vi "Dashboard Main.vi"() -> ()   [LabVIEW 2016]
uses:
  <vilib>/Utility/miscctls.llb/LVRowAndColumnTypeDef.ctl
  <vilib>/event_ctls.llb/eventvkey.ctl
  <vilib>/Rock Robotics/Network Tables/NT Read Numeric Array.vi
  <vilib>/Rock Robotics/Network Tables/NT Write Boolean.vi
  <vilib>/Rock Robotics/WPI/Dashboard/WPI_DashboardLogging Global.vi
panel:
  out "Camera Info 2":cluster{"Mbps LED":bool, "Mbps":dbl, "fps":dbl} {"fps" format="%#.1g"; "Mbps" format="%#.1g"}
  out "Background":bool
  out "Camera Image Right":T1(plugin-control)
  in  "Camera Settings Right":T2={"Frame Rate"=30, "Compression"=30, "Size"=1, "DB Camera Config"=FALSE} {"Frame Rate" scale=1.0..30.0; "Compression" scale=100.0..-1.0; "Size" items=["640x480", "320x240", "160x120"]}
  in  "Camera Name Right":string(combo)="No Camera Selection"
  out "Camera Info":cluster{"Mbps LED":bool, "Mbps":dbl, "fps":dbl} {"fps" format="%#.1g"; "Mbps" format="%#.1g"}
  in  "Camera Settings":T2={"Frame Rate"=30, "Compression"=30, "Size"=1, "DB Camera Config"=FALSE} {"Frame Rate" scale=1.0..30.0; "Compression" scale=100.0..-1.0; "Size" items=["640x480", "320x240", "160x120"]}
  in  "TCP":refnum<k5>
  in  "Rec Mode":enum32{"Stop", "Record", "Playback"}(radio)
  out "Robot IP":string
  out "Image Message":string="Timeout in Camera Communications"
  in  "Dashboard Tab":T3(tab)
  out "GEAR POSITION":string
  in  "Select Auto":string(combo)="Select Autonomous ..."
  out "NT Connection":bool
  out "MotorChart R":cluster{"Numeric":dbl, "Numeric":dbl}(graph)
  out "MotorChart L":cluster{"Numeric":dbl, "Numeric":dbl}(graph)
  out "MotorSliders R":cluster{"MotorSlide1":dbl, "MotorSlide2":dbl} {"MotorSlide2" scale=-1.0..1.0 scale format="%#_2e"; "MotorSlide1" scale=-1.0..1.0 scale format="%#_2e"}
  out "MotorSliders L":cluster{"MotorSlide1":dbl, "MotorSlide2":dbl} {"MotorSlide2" scale=-1.0..1.0 scale format="%#_2e"; "MotorSlide1" scale=-1.0..1.0 scale format="%#_2e"}
  out "Gyro":dbl(knob) scale=0.0..360.0
  out "JS1 Z":dbl(slide) scale=-1.0..1.0 scale format="%#_2e"
  out "JS1 Graph":cluster{"X":dbl, "Y":dbl}[](graph)
  out "JS1 Buttons":T4
  out "JS2 Z":dbl(slide) scale=-1.0..1.0 scale format="%#_2e"
  out "JS2 Graph":cluster{"X":dbl, "Y":dbl}[](graph)
  out "JS2 Buttons":T4
  out "Mode":T5(ring)=enum."Auto Disabled"
  in  "Drive Inverter":bool=TRUE
  in  "Turn Angle Target":dbl=30.0
  out "GEAR POSITION":dbl format="%#_13g"
  in  "Slow Speed":dbl(slide)=0.49999999999999994 scale=0.0..1.0
  out "Gyro Raw":dbl
  out "X-Axis Value":dbl=3.0 format="%#_13g"
  in  "D":dbl
  in  "I":dbl=10.0
  in  "Low":dbl=0.8
  in  "P":dbl=0.3
  in  "High":dbl=0.8
  in  "DB/String 9":string
  in  "DB/String 8":string
  in  "DB/String 7":string
  in  "DB/String 6":string
  in  "DB/String 5":string
  in  "DB/String 4":string
  in  "DB/String 3":string
  in  "DB/String 2":string
  in  "DB/String 1":string
  in  "DB/String 0":string
  in  "DB/Slider 0":dbl(slide) scale=0.0..5.0
  in  "DB/Slider 1":dbl(slide) scale=0.0..5.0
  in  "DB/Slider 2":dbl(slide) scale=0.0..5.0
  in  "DB/Slider 3":dbl(slide) scale=0.0..5.0
  out "DB/LED 3":bool
  out "DB/LED 2":bool
  out "DB/LED 1":bool
  out "DB/LED 0":bool
  in  "DB/Button 3":bool
  in  "DB/Button 2":bool
  in  "DB/Button 1":bool
  in  "DB/Button 0":bool caption="New Name"
  out "X-Axis Chart":dbl(graph)
  in  "T3":dbl=5.0
  in  "T2":dbl=2.0
  in  "T1":dbl=5.0
  in  "Y2":dbl=0.8
  in  "Y1":dbl=0.8
  in  "T4":dbl=3.0
  in  "X":dbl=-0.32
  in  "Y":dbl=0.8
  in  "Time":dbl=1.25
  in  "Gear Time":dbl=4.0
  in  "Time":dbl=1.0
  in  "Y 2":dbl=0.6
  in  "X 2":dbl=-0.32
  in  "Test Slider":dbl(slide) scale=0.0..100.0 scale format="%#_3g"
  in  "On/Off":bool caption="Solenoid"
  in  "Test Name":u16(ring) items=["Select the test to run..."]
  in  "Test Tree":string(tree)
  in  "Motor":cluster{"Value":dbl, "Enable":bool} {"Value" scale=-1.0..1.0 scale format="%#_3g"}
  out "Progress":T6 {"Test Progress" scale=0.0..100.0}
  in  "Rev/Fwd":cluster{"Forward":bool, "Reverse":bool}
  in  "Test Ring":u16(ring) items=["Monochrome", "Color"]
  out "Cmd Status":string
  in  "Execute Command":bool
  in  "Command Params":string[][](table)
  in  "Command Selection":i32(listbox)
  in  "CheckList":i32(listbox)
  out "Tree":string(tree)
  out "Camera Image":T1(plugin-control)
  in  "Camera Name":string(combo)="No Camera Selection"
  # "HW"
  # "HW"
  # "Joysticks"
  # "Drive Motors"
  # "Front"
  # "Right"
  # "Left"
  # "Back"
  # "POSITION 3 AUTON"
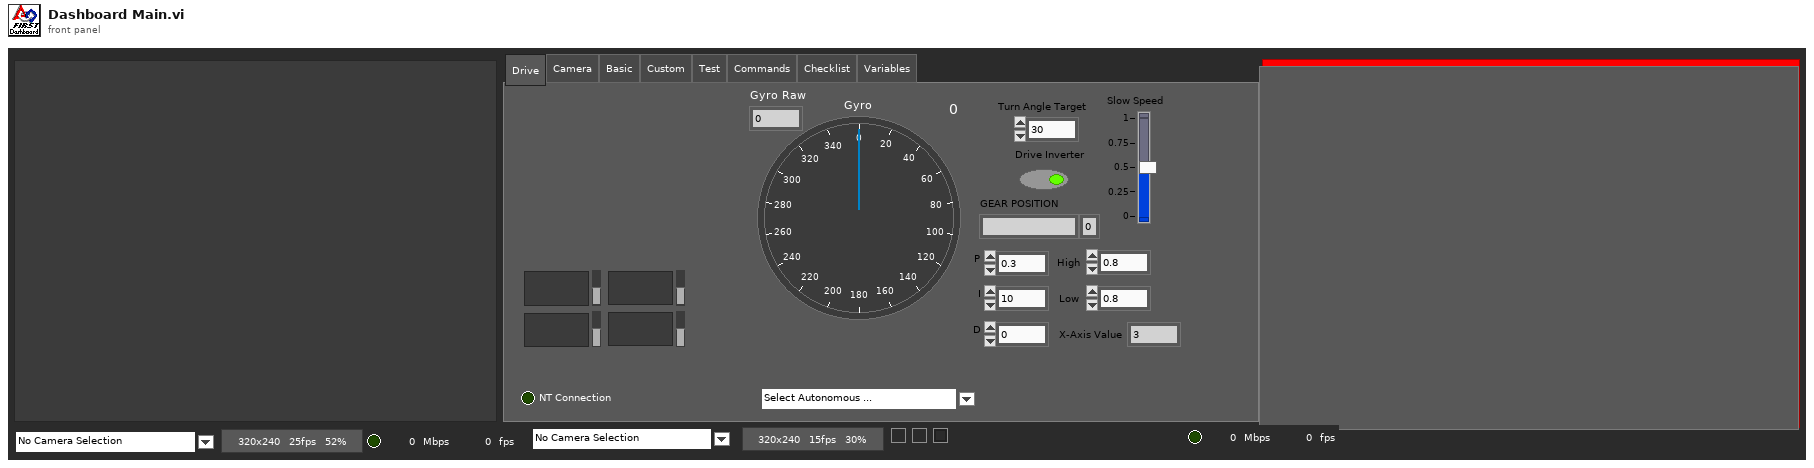
[diagram p1: front panel]
types:
  T1 = typedef "IMAQ Image.ctl" = refnum<image>
  T2 = cluster{"Frame Rate":i32, "Compression":i32, "Size":u16, "DB Camera Config":bool}
  T3 = enum32{"Drive", "Camera", "Basic", "Custom", "Test", "Commands", "Checklist", "Variables"}
  T4 = cluster{bool, bool, bool, bool, bool, bool, bool, bool, bool, bool, bool, bool}
  T5 = enum8{"Tele-Op Disabled", "Tele-Op Enabled", "Auto Disabled", "Auto Enabled", "Test Disabled", "Test Enabled", "Disconnected", "No Code", "E-Stop"}
  T6 = cluster{"Test Progress":u8, "Test Progress Text":string}
  T7 = typedef "Image Type" = u32
  T8 = cluster{"IDs":cluster{"RPC field ID":u16, "Unique ID":u16}, "String":string}
  T9 = enum32{"Drive", "Basic", "Custom", "Test", "Checklist", "Variables"}
  T10 = cluster{"Camera Image":refnum<vi>, "Dashboard Tab":refnum<vi>, "Background":refnum<vi>, "Rec Mode":refnum<vi>, "Test Slider":refnum<vi>, "On/Off ":refnum<vi>, "Test Ring":refnum<vi>, "Rev/Fwd":refnum<vi>, "Test Name":refnum<vi>, "Motor":refnum<vi>, "Progress":refnum<vi>, "CheckList":refnum<vi>, "Tree":refnum<vi>, "Test Tree":refnum<vi>, "Command Params":refnum<vi>, "Command Selection":refnum<vi>, "Execute Command":refnum<vi>, "Cmd Status":refnum<vi>, "Camera Settings":refnum<vi>, "Camera Name":refnum<vi>, "Camera Info":refnum<vi>, "Camera Settings Right":refnum<vi>, "Camera Name Right":refnum<vi>, "Camera Image Right":refnum<vi>}
  T11 = cluster{"Error Strings":string, "Disable Counts":cluster{u16, u16}, "Rail Faults":cluster{u16, u16, u16}, "Robot IP":string, "DB Mode":u8, "Event Info":cluster{"Name":string, "Type":u8, "Number":u16, "Replay":u8}}
  T12 = cluster{"Storage":cluster{"Disk Free":u64, "RAM Block":u32, "RAM free":u32}, "CPU Utilization":cluster{"CPU % ISR":sgl, "CPU % Time Crit":sgl, "CPU % Timed Str":sgl, "CPU % High":sgl, "CPU % Above":sgl, "CPU % Normal":sgl, "CPU % Low":sgl}, "CAN":cluster{"% Bus Utilization":sgl, "Bus Off Cnt":u32, "TX_FIFO Full Cnt":u32, "Receive Error Cnt":u8, "Transmit Error Cnt":u8}, "HID":cluster{"HID Outputs":u32, "Rumble Low":u16, "Rumble High":u16}[]}
  T13 = cluster{"Status bits":cluster{"Test Mode":bool, "Autonomous":bool, "Enabled":bool, "Code Start":bool, "Brownout":bool, "Reserved 2":bool, "Reserved 3":bool, "E-Stop":bool}, "Code Trace":cluster{"Disabled":bool, "TeleOp":bool, "Auto":bool, "Test":bool}, "Controller Type":enum16{"unknown", "cRIO", "roboRio"}, "Code?":enum16{"unknown", "noCode", "code"}, "Battery V":dbl}
  T14 = cluster{"Control Bits":cluster{"TestMode":bool, "Autonomous":bool, "Enabled":bool, "FMS Present":bool, bool, bool, bool, "E-Stop":bool}, "Team Station ":u8, "Countdown":sgl, "Joystick Values":cluster{"Axes":dbl[], "Buttons":bool[], "POVs":i16[]}[]}
  T15 = cluster{"Axes":dbl[], "Buttons":bool[], "POVs":i16[]}[]
  T16 = cluster{"Axes":dbl[], "Buttons":bool[], "POVs":i16[]}
  T17 = cluster{"Buttons[0]":bool, "Buttons[1]":bool, "Buttons[2]":bool, "Buttons[3]":bool, "Buttons[4]":bool, "Buttons[5]":bool, "Buttons[6]":bool, "Buttons[7]":bool, "Buttons[8]":bool, "Buttons[9]":bool, "Buttons[10]":bool, "Buttons[11]":bool}
  T18 = cluster{"Operation":enum16{"Update", "Clear"}, "Color Box":u32}[]
  T19 = typedef "eventvkey.ctl" = enum16{"ASCII", "Enter", "Return", "Shift", "Ctrl", "Alt", "Cmd", "Opt", "Caps", "NumLock", "Clear", "Break", "Up", "Down", "Left", "Right", "Insert", "Delete", "Home", "End", "PageUp", "PageDown", "Escape", "Help", "Pause", "ScrollLock", "F1", "F2", "F3", "F4", "F5", "F6", "F7", "F8", "F9", "F10", "F11", "F12", "F13", "F14", "F15", "F16", "F17", "F18", "F19", "F20", "F21", "F22", "F23", "F24", "Play", "VolumeUp", "VolumeDown", "Mute", "Two Byte Char"}
  T20 = cluster{"Image Size":bool, "Image Type":bool, "Pixel Value":bool, "ROI Information":bool, "Zoom Factor":bool}
  T21 = cluster{"Operation":enum16{"Update", "Clear"}, "Color Box":u32}
  T22 = typedef "LVRowAndColumnTypeDef.ctl" = cluster{"Row":i32, "Column":i32}
  T23 = cluster{"Shift":bool, "Ctrl":bool, "Alt":bool, "Cmd":bool, "Opt":bool}
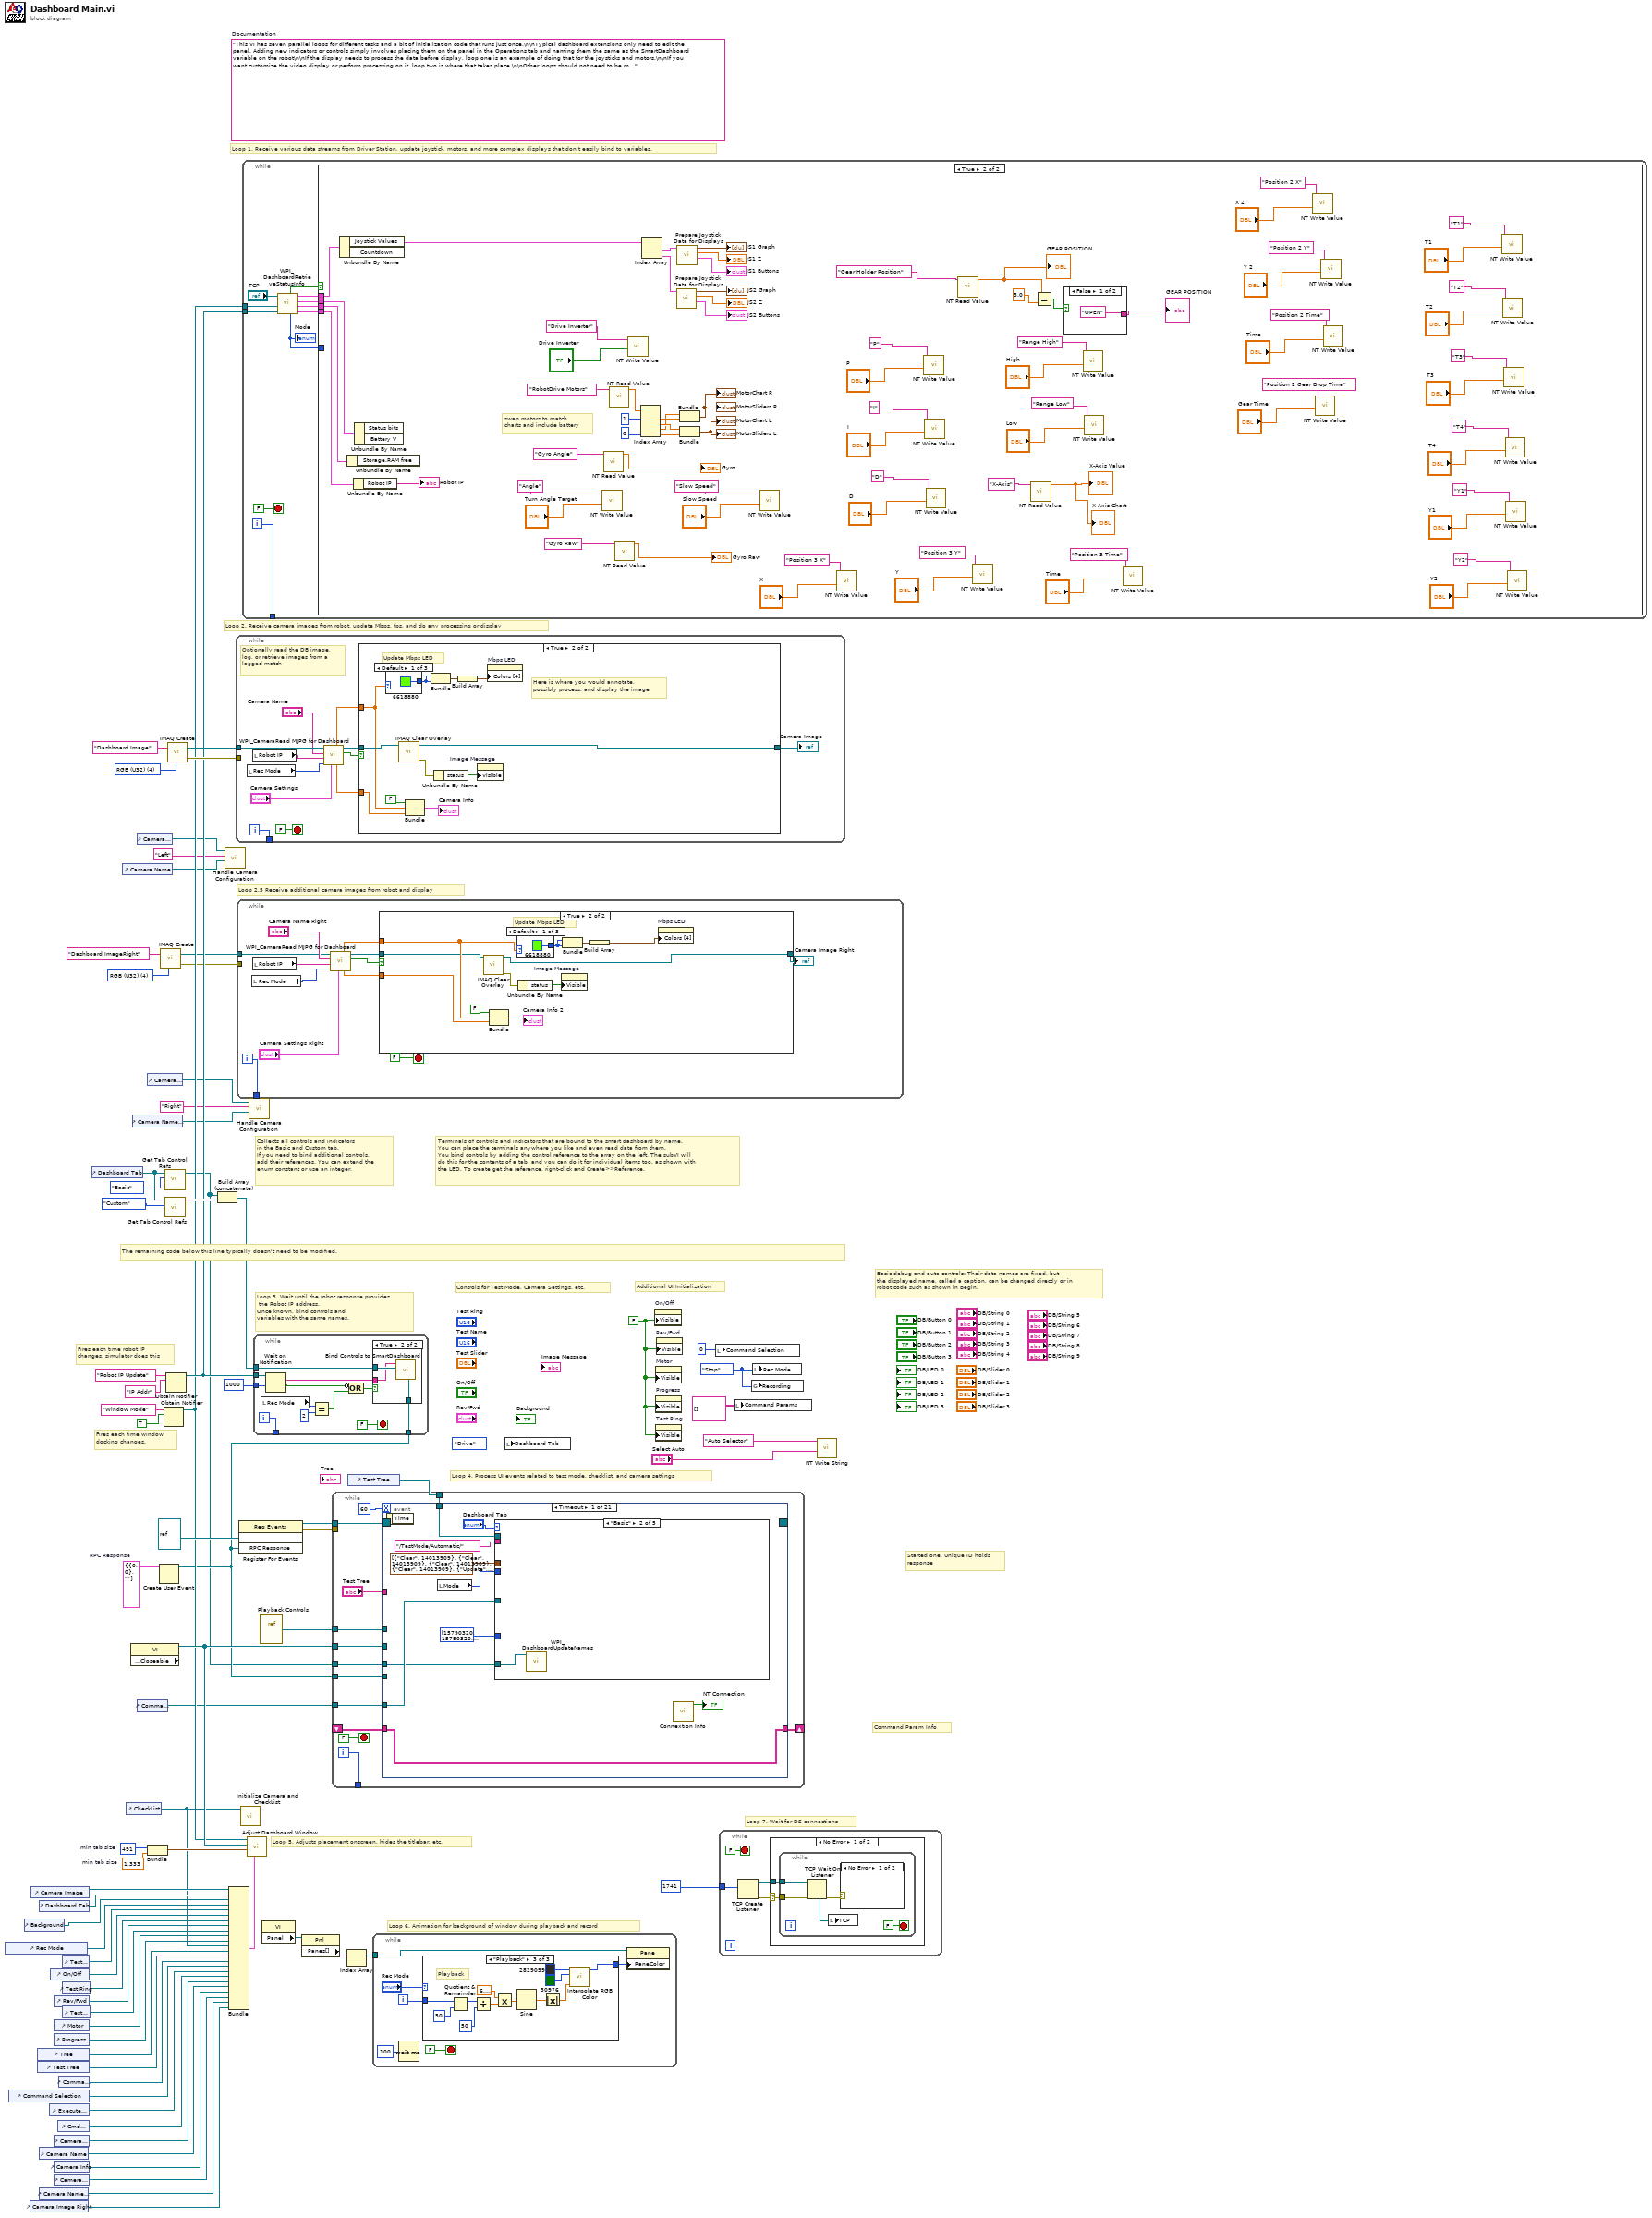
[diagram p0: block diagram]
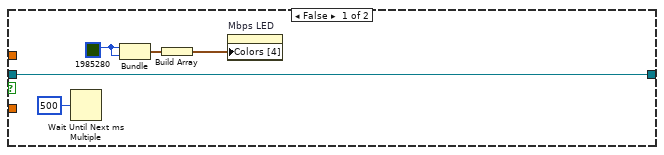
[diagram p2: hidden frame]
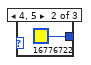
[diagram p3: hidden frame]
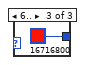
[diagram p4: hidden frame]
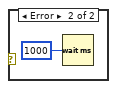
[diagram p5: hidden frame]
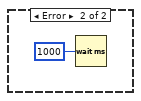
[diagram p6: hidden frame]
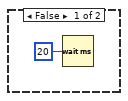
[diagram p7: hidden frame]
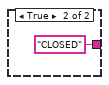
[diagram p8: hidden frame]
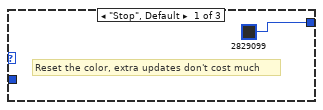
[diagram p9: hidden frame]
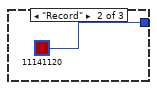
[diagram p10: hidden frame]
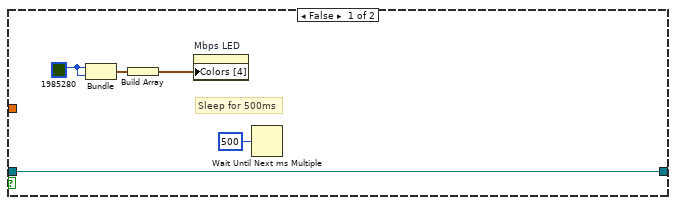
[diagram p12: hidden frame]
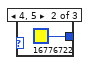
[diagram p13: hidden frame]
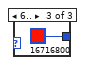
[diagram p14: hidden frame]
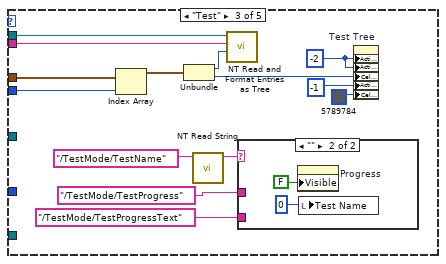
[diagram p16: hidden frame]
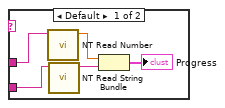
[diagram p17: hidden frame]
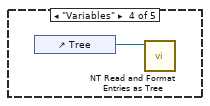
[diagram p18: hidden frame]
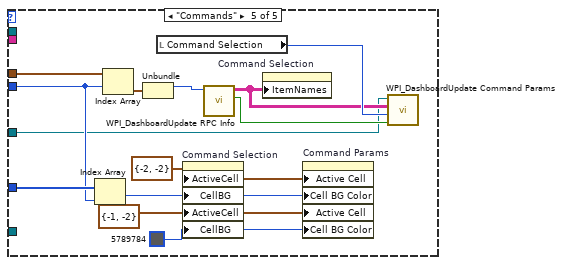
[diagram p19: hidden frame]
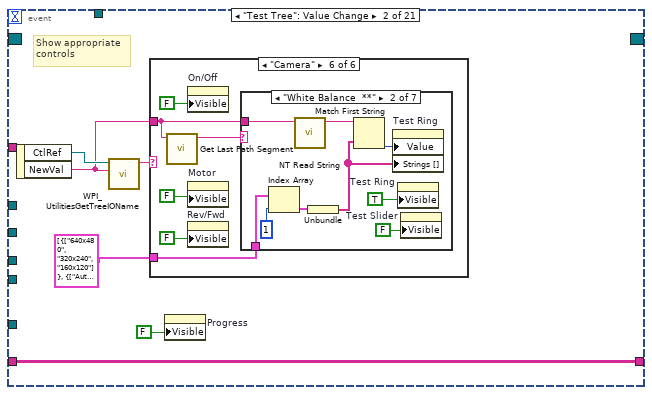
[diagram p20: hidden frame]
diagram:
  w12 = T7 4 items=["Grayscale (U8)", "Grayscale (I16)", "Grayscale (SGL)", "Complex (CSG)", "RGB (U32)", "HSL (U32)", "RGB (U64)"] ("Image Type")
  w28 = T8 {"IDs"={"RPC field ID"=0, "Unique ID"=0}, "String"=""}  # RPC Response
  w51 = 491  # min tab size
  w50 = 1.333  # min tab size
  w58 = enum32{"Stop", "Record", "Playback"}."Stop" ("Rec Mode")
  w34 = FALSE ("Visible")
  (unwired) "This VI has seven parallel loops for different tasks and a bit of initialization code that runs just once.\n\nTypical dashboard extensions only need to edit the panel. Adding new indicators or controls simply involves placing them on the panel in the Operations tab and naming them the same as the SmartDashboard variable on the robot\n\nIf the display needs to process the data before display, loop one is an example of doing that for the joysticks and motors.\n\nIf you want customize the video display or perform processing on it, loop two is where that takes place.\n\nOther loops should not need to be modified. They are pretty standard, and document the task they perform."  # Documentation
  w75 = T7 4 items=["Grayscale (U8)", "Grayscale (I16)", "Grayscale (SGL)", "Complex (CSG)", "RGB (U32)", "HSL (U32)", "RGB (U64)"] ("Image Type")
  # "Loop 2.5 Receive additional camera images from robot and display"
  # "Command Param Info"
  # "Started one, Unique ID holds\nresponse"
  # "Loop 7. Wait for DS connections"
  # "Basic debug and auto controls: Their data names are fixed, but\nthe displayed name, called a caption, can be changed directly or in\nrobot code such as shown in Begin."
  # "Controls for Test Mode, Camera Settings, etc."
  # "Additional UI Initialization"
  # "Loop 6. Animation for background of window during playback and record"
  # "Fires each time robot IP\nchanges, simulator does this"
  # "Fires each time window\ndocking changes."
  # "Collects all controls and indicators\nin the Basic and Custom tab.\nIf you need to bind additional controls,\nadd their references. You can extend the\nenum constant or use an integer."
  # "The remaining code below this line typically doesn't need to be modified."
  # "Loop 4. Process UI events related to test mode, checklist, and camera settings"
  # "Terminals of controls and indicators that are bound to the smart dashboard by name.\nYou can place the terminals anywhere you like and even read data from them.\nYou bind controls by adding the control reference to the array on the left. The subVI will\ndo this for the contents of a tab, and you can do it for individual items too, as shown with\nthe LED. To create get the reference, right-click and Create>>Reference."
  # "Loop 3. Wait until the robot response provides\n the Robot IP address.\nOnce known, bind controls and\nvariables with the same names."
  # "Loop 5. Adjusts placement onscreen, hides the titlebar, etc."
  # "Loop 1. Receive various data streams from Driver Station, update joystick, motors, and more complex displays that don't easily bind to variables."
  # "Loop 2. Receive camera images from robot, update Mbps, fps, and do any processing or display"
  n1 = control-ref of="Rec Mode"() -> (w40:refnum<vi>)
  n2 = control-ref of="Command Selection"() -> (w27:refnum<vi>)
  n3 = control-ref of="Background"() -> (w1:refnum<vi>)
  n4 = control-ref of="Camera Image Right"() -> (w3:refnum<vi>)
  n5 = control-ref of="Camera Image"() -> (w53:refnum<vi>)
  n6 = control-ref of="Tree"() -> (w44:refnum<vi>)
  n7 = control-ref of="Test Tree"() -> (w43:refnum<vi>)
  n8 = control-ref of="Dashboard Tab"() -> (w52:refnum<vi>)
  n9 = control-ref of="Camera Name"() -> (w18:refnum<vi>)
  n10 = control-ref of="Camera Name Right"() -> (w4:refnum<vi>)
  n11 = control-ref of="Execute Command"() -> (w29:refnum<vi>)
  n12 = control-ref of="On/Off"() -> (w38:refnum<vi>)
  n13 = control-ref of="Progress"() -> (w35:refnum<vi>)
  n14 = control-ref of="Camera Settings"() -> (w19:refnum<vi>)
  n15 = control-ref of="Camera Info"() -> (w17:refnum<vi>)
  n16 = control-ref of="Camera Settings Right"() -> (w5:refnum<vi>)
  n17 = control-ref of="Rev/Fwd"() -> (w36:refnum<vi>)
  n18 = control-ref of="Motor"() -> (w41:refnum<vi>)
  n19 = control-ref of="Cmd Status"() -> (w23:refnum<vi>)
  n20 = control-ref of="Command Params"() -> (w30:refnum<vi>)
  n21 = control-ref of="Test Slider"() -> (w39:refnum<vi>)
  n22 = control-ref of="Test Ring"() -> (w37:refnum<vi>)
  n23 = control-ref of="Test Name"() -> (w42:refnum<vi>)
  n24 = control-ref of="Dashboard Tab"() -> (w56:refnum<vi>)
  n25 = control-ref of="Camera Name"() -> (w20:refnum<vi>)
  n26 = control-ref of="CheckList"() -> (w45:refnum<vi>)
  n27 = property class="VI" props=["Front Panel.Closeable"]() -> (reference out=w57:refnum<vi>)  [unwired: 2 in, 2 out]
  n28 = control-ref of="Camera Name Right"() -> (w8:refnum<vi>)
  n29 = control-ref of="Camera Settings"() -> (w21:refnum<vi>)
  n30 = control-ref of="Command Params"() -> (w22:refnum<vi>)
  n31 = control-ref of="Camera Settings Right"() -> (w9:refnum<vi>)
  n32 = Bundle("min tab size"=w51, "min tab size"=w50) -> (w49:cluster{"min tab size":i32, "min tab size":dbl})  [unwired: 1 in]
  n33 = Create User Event(user event datatype=w28) -> (user event=w24:refnum<user-event>)  [unwired: 1 in, 1 out]
  n34 = call "IMAQ Create"("Image Name"="Dashboard ImageRight", "Image Type"=w12) -> ("New Image"=w11:T1, "error out"=w10:errorcluster)  [unwired: 2 in, 1 out]
  n35 = Obtain Notifier(name (unnamed)="Window Mode", notification data type=TRUE) -> (notifier out=w32:refnum<notifier>)  [unwired: 2 in, 2 out]
  n36 = call <vilib>:"Get Tab Control Refs.vi"("Page Index"=T9."Basic" ("Dashboard Tab"), "TabControl in"=w56) -> ("ControlsOnPage"=w16:refnum<vi>[])  [unwired: 9 in]
  n37 = call <vilib>:"Get Tab Control Refs.vi"("Page Index"=T9."Custom" ("Dashboard Tab"), "TabControl in"=w56) -> ("ControlsOnPage"=w55:refnum<vi>[])  [unwired: 9 in]
  n38 = Obtain Notifier(name (unnamed)="Robot IP Update", notification data type="IP Addr" ("name (unnamed)")) -> (notifier out=w33:refnum<notifier>)  [unwired: 2 in, 2 out]
  n39 = call "IMAQ Create"("Image Name"="Dashboard Image", "Image Type"=w75) -> ("New Image"=w73:T1, "error out"=w72:errorcluster)  [unwired: 2 in, 1 out]
  n40 = Build Array (concatenate)(w16, w55) -> (w54:refnum<vi>[])
  n41 = call "Handle Camera Configuration.vi"("CameraNameRef"=w20, "Camera File Name"="Left", "ClusterRef"=w21) -> ()  [unwired: 9 in]
  n42 = Bundle("Camera Image"=w53, "Dashboard Tab"=w52, "Background"=w1, "Rec Mode"=w40, "Test Slider"=w39, "On/Off"=w38, "Test Ring"=w37, "Rev/Fwd"=w36, "Test Name"=w42, "Motor"=w41, "Progress"=w35, "CheckList"=w45, "Tree"=w44, "Test Tree"=w43, "Command Params"=w30, "Command Selection"=w27, "Execute Command"=w29, "Cmd Status"=w23, "Camera Settings"=w19, "Camera Name"=w18, "Camera Info"=w17, "Camera Settings Right"=w5, "Camera Name Right"=w4, "Camera Image Right"=w3) -> (w46:T10)  [unwired: 1 in]
  n43 = while {
    tunnel: w73 -> [w85]
    tunnel: w72 -> [_]
    tunnel: [w86] -> _
    i -> [w86]
    stop <- FALSE stop-if-true
    # "Optionally read the DB image,\nlog, or retrieve images from a\nlogged match"
    n44 = local read "Rec Mode"() -> (w81:enum32{"Stop", "Record", "Playback"})
    n45 = local read "Robot IP"() -> (w80:string)
    n46 = call <vilib>:"WPI_CameraRead MJPG for Dashboard.vi"("Camera Settings"="Camera Settings", "Rec Mode"=w81, "Robot IP"=w80, "Camera Name"="Camera Name", "Refnum in"=w85) -> ("Active"=w83:bool, "Refnum out"=w84:T1, "FPS"=w82:dbl, "Bandwidth (Mbps)"=w79:dbl)  [unwired: 3 in]
    n47 = case shown="True" w83 {
      tunnel: w84 -> [w88 w99]
      tunnel: w79 -> [_ w96]
      tunnel: w82 -> [_ w97]
      tunnel: [w88 w93] -> w76
      frame False {
        w90 = u32 1985280 ("Color Box")
        # "Sleep for 500ms"
        n48 = Bundle("Color Box"=w90, "Color Box"=w90) -> (w91:cluster{"Color Box":u32, "Color Box":u32})  [unwired: 1 out]
        n49 = Build Array(w91) -> (w89:cluster{"Color Box":u32, "Color Box":u32}[])
        n50 = property on="Mbps LED" class="Bool (strict)"("Colors [4]"=w89) -> ()  [unwired: 2 in, 2 out]
        n51 = Wait Until Next ms Multiple(millisecond multiple=u32 500) -> ()  [unwired: 1 out]
      }
      frame True {
        # "Here is where you would annotate,\npossibly process, and display the image"
        # "Update Mbps LED"
        n52 = case shown="Default" w96 {
          tunnel: [u32 6618880 ("Color Box") u32 16776722 ("Color Box") u32 16716800 ("Color Box")] -> w100
          frame Default {
          }
          frame 4, 5 {
          }
          frame 6.. {
          }
        }
        n53 = call "IMAQ Clear Overlay"("Image"=w99) -> ("error out"=w102:errorcluster, "Image Out"=w93:T1)  [unwired: 2 in, 7 out]
        n54 = Bundle(FALSE, "Bandwidth (Mbps)"=w96, "FPS"=w97) -> (→"Camera Info":cluster{bool, "Bandwidth (Mbps)":dbl, "FPS":dbl})  [unwired: 1 in]
        n55 = Bundle("Color Box"=w100, "Color Box"=w100) -> (w101:cluster{"Color Box":u32, "Color Box":u32})  [unwired: 1 out]
        n56 = Unbundle By Name(w102) -> ("status"=w103:bool)
        n57 = Build Array(w101) -> (w98:cluster{"Color Box":u32, "Color Box":u32}[])
        n58 = property on="Image Message" class="Str"("Visible"=w103) -> ()  [unwired: 2 in, 2 out]
        n59 = property on="Mbps LED" class="Bool (strict)"("Colors [4]"=w98) -> ()  [unwired: 2 in, 2 out]
      }
    }
    "Camera Image" <- w76
  }
  n60 = while {
    tunnel: w11 -> [w117]
    tunnel: w10 -> [_]
    tunnel: [w111] -> _
    i -> [w111]
    stop <- FALSE stop-if-true
    n61 = local read "Rec Mode"() -> (w115:enum32{"Stop", "Record", "Playback"})
    n62 = local read "Robot IP"() -> (w116:string)
    n63 = call <vilib>:"WPI_CameraRead MJPG for Dashboard.vi"("Camera Settings"="Camera Settings Right", "Rec Mode"=w115, "Robot IP"=w116, "Camera Name"="Camera Name Right", "Refnum in"=w117) -> ("Active"=w110:bool, "Refnum out"=w113:T1, "FPS"=w108:dbl, "Bandwidth (Mbps)"=w109:dbl)  [unwired: 3 in]
    n64 = case shown="True" w110 {
      tunnel: w113 -> [w122 w125]
      tunnel: w109 -> [_ w127]
      tunnel: w108 -> [_ w130]
      tunnel: [w122 w124] -> w107
      frame False {
        w120 = u32 1985280 ("Color Box")
        n65 = Wait Until Next ms Multiple(millisecond multiple=u32 500) -> ()  [unwired: 1 out]
        n66 = Bundle("Color Box"=w120, "Color Box"=w120) -> (w119:cluster{"Color Box":u32, "Color Box":u32})  [unwired: 1 out]
        n67 = Build Array(w119) -> (w121:cluster{"Color Box":u32, "Color Box":u32}[])
        n68 = property on="Mbps LED" class="Bool (strict)"("Colors [4]"=w121) -> ()  [unwired: 2 in, 2 out]
      }
      frame True {
        # "Update Mbps LED"
        n69 = call "IMAQ Clear Overlay"("Image"=w125) -> ("error out"=w132:errorcluster, "Image Out"=w124:T1)  [unwired: 2 in, 7 out]
        n70 = Bundle(FALSE, "Bandwidth (Mbps)"=w127, "FPS"=w130) -> (→"Camera Info 2":cluster{bool, "Bandwidth (Mbps)":dbl, "FPS":dbl})  [unwired: 1 in]
        n71 = case shown="Default" w127 {
          tunnel: [u32 6618880 ("Color Box") u32 16776722 ("Color Box") u32 16716800 ("Color Box")] -> w128
          frame Default {
          }
          frame 4, 5 {
          }
          frame 6.. {
          }
        }
        n72 = Unbundle By Name(w132) -> ("status"=w131:bool)
        n73 = property on="Image Message" class="Str"("Visible"=w131) -> ()  [unwired: 2 in, 2 out]
        n74 = Bundle("Color Box"=w128, "Color Box"=w128) -> (w129:cluster{"Color Box":u32, "Color Box":u32})  [unwired: 1 out]
        n75 = Build Array(w129) -> (w126:cluster{"Color Box":u32, "Color Box":u32}[])
        n76 = property on="Mbps LED" class="Bool (strict)"("Colors [4]"=w126) -> ()  [unwired: 2 in, 2 out]
      }
    }
    "Camera Image Right" <- w107
  }
  n77 = register-events(refnum<vi> refnum, w24) -> (reference out=w62:refnum<event-registration>, error out=w61:errorcluster)  [unwired: 2 in]
  n78 = call "Initialize Camera and CheckList.vi"("ListBox in"=w45) -> ()  [unwired: 11 in]
  n79 = while {
    tunnel: [w147] -> _
    tunnel: w33 -> [w141]
    tunnel: w32 -> [w138]
    i -> [w147]
    stop <- FALSE stop-if-true
    n80 = call <vilib>:"WPI_DashboardRetrieveStatusInfo.vi"("Binding Refnum"=w141, "Window Mode Notifier"=w138, "TCP Cnx"="TCP") -> ("Power and Errors"=w142:T11, "Robot Metrics"=w145:T12, "Status Info"=w146:T13, "Control Info"=w143:T14, "Robot Mode"=w140:T5, "Process?"=w144:bool)  [unwired: 3 in]
    "Mode" <- w140
    n81 = case shown="True" w144 {
      tunnel: w146 -> [_ w226]
      tunnel: w145 -> [_ w225]
      tunnel: w143 -> [_ w224]
      tunnel: w142 -> [_ w223]
      tunnel: w140 -> [_ _]
      frame False {
        n82 = Wait (ms)(milliseconds to wait=u32 20) -> ()  [unwired: 1 out]
      }
      frame True {
        # "swap motors to match\ncharts and include battery"
        n83 = Unbundle By Name(w224) -> ("Joystick Values"=w214:T15)  [unwired: 1 out]
        n84 = Unbundle By Name(w225) -> ()  [unwired: 1 out]
        n85 = Unbundle By Name(w223) -> ("Robot IP"=→"Robot IP":string)
        n86 = Unbundle By Name(w226) -> ()  [unwired: 2 out]
        n87 = call-poly <vilib>:"NT Write Value.vi"("Numeric"="Turn Angle Target", "Name"="Angle") -> ()  [unwired: 9 in, 1 out]
        n88 = call-poly <vilib>:"NT Read Value.vi"("Name"="Gyro Angle") -> ("Numeric"=→"Gyro":dbl)  [unwired: 9 in, 1 out]
        n89 = call-poly <vilib>:"NT Read Value.vi"("Name"="RobotDrive Motors") -> ("Numeric Array"=w204:dbl[])  [unwired: 9 in, 1 out]
        n90 = call-poly <vilib>:"NT Read Value.vi"("Name"="Gyro Raw") -> ("Numeric"=→"Gyro Raw":dbl)  [unwired: 9 in, 1 out]
        n91 = call-poly <vilib>:"NT Write Value.vi"("Boolean"="Drive Inverter", "Name"="Drive Inverter" ("refnum name")) -> ()  [unwired: 9 in, 1 out]
        n92 = Index Array(array=w204, index #1=1, index #4=0) -> (element #1=w218:dbl, element #2=w219:dbl, element #3=w217:dbl, element #4=w222:dbl)  [unwired: 2 in]
        n93 = Index Array(array=w214) -> (element #1=w213:T16, element #2=w209:T16)  [unwired: 2 in]
        n94 = call "Prepare Joystick Data for Displays.vi"("Joystick Values"=w209) -> ("Buttons"=→"JS2 Buttons":T17, "Z Axis"=→"JS2 Z":dbl, "Cartesian Data"=→"JS2 Graph":cluster{"X axis":dbl, "X axis":dbl}[])  [unwired: 8 in]
        n95 = call "Prepare Joystick Data for Displays.vi"("Joystick Values"=w213) -> ("Buttons"=→"JS1 Buttons":T17, "Z Axis"=→"JS1 Z":dbl, "Cartesian Data"=→"JS1 Graph":cluster{"X axis":dbl, "X axis":dbl}[])  [unwired: 8 in]
        n96 = Bundle("Numeric"=w217, "Numeric"=w218) -> (→"MotorChart R" →"MotorSliders R":cluster{"Numeric":dbl, "Numeric":dbl})  [unwired: 1 in]
        n97 = Bundle("Numeric"=w219, "Numeric"=w222) -> (→"MotorChart L" →"MotorSliders L":cluster{"Numeric":dbl, "Numeric":dbl})  [unwired: 1 in]
        n98 = call-poly <vilib>:"NT Write Value.vi"("Numeric"="Slow Speed", "Name"="Slow Speed") -> ()  [unwired: 9 in, 1 out]
        n99 = call-poly <vilib>:"NT Write Value.vi"("Numeric"="X", "Name"="Position 3 X") -> ()  [unwired: 9 in, 1 out]
        n100 = call-poly <vilib>:"NT Write Value.vi"("Numeric"="P", "Name"="P") -> ()  [unwired: 9 in, 1 out]
        n101 = call-poly <vilib>:"NT Write Value.vi"("Numeric"="I", "Name"="I") -> ()  [unwired: 9 in, 1 out]
        n102 = call-poly <vilib>:"NT Write Value.vi"("Numeric"="D", "Name"="D") -> ()  [unwired: 9 in, 1 out]
        n103 = call-poly <vilib>:"NT Read Value.vi"("Name"="Gear Holder Position") -> ("Numeric"=w194:dbl)  [unwired: 9 in, 1 out]
        "GEAR POSITION" <- w194
        n104 = call-poly <vilib>:"NT Write Value.vi"("Numeric"="Y", "Name"="Position 3 Y") -> ()  [unwired: 9 in, 1 out]
        n105 = call-poly <vilib>:"NT Read Value.vi"("Name"="X-Axis") -> ("Numeric"=→"X-Axis Value" →"X-Axis Chart":dbl)  [unwired: 9 in, 1 out]
        n106 = Equal?(x=w194, y=3.0) -> (x = y?=w193:bool)
        n107 = case shown="False" w193 {
          tunnel: ["OPEN" "CLOSED"] -> w192
          frame False {
          }
          frame True {
          }
        }
        "GEAR POSITION" <- w192
        n108 = call-poly <vilib>:"NT Write Value.vi"("Numeric"="High", "Name"="Range High") -> ()  [unwired: 9 in, 1 out]
        n109 = call-poly <vilib>:"NT Write Value.vi"("Numeric"="Low", "Name"="Range Low") -> ()  [unwired: 9 in, 1 out]
        n110 = call-poly <vilib>:"NT Write Value.vi"("Numeric"="Time", "Name"="Position 3 Time") -> ()  [unwired: 9 in, 1 out]
        n111 = call-poly <vilib>:"NT Write Value.vi"("Numeric"="X 2", "Name"="Position 2 X") -> ()  [unwired: 9 in, 1 out]
        n112 = call-poly <vilib>:"NT Write Value.vi"("Numeric"="Gear Time", "Name"="Position 2 Gear Drop Time") -> ()  [unwired: 9 in, 1 out]
        n113 = call-poly <vilib>:"NT Write Value.vi"("Numeric"="Y 2", "Name"="Position 2 Y") -> ()  [unwired: 9 in, 1 out]
        n114 = call-poly <vilib>:"NT Write Value.vi"("Numeric"="Time", "Name"="Position 2 Time") -> ()  [unwired: 9 in, 1 out]
        n115 = call-poly <vilib>:"NT Write Value.vi"("Numeric"="T1", "Name"="T1") -> ()  [unwired: 9 in, 1 out]
        n116 = call-poly <vilib>:"NT Write Value.vi"("Numeric"="T2", "Name"="T2") -> ()  [unwired: 9 in, 1 out]
        n117 = call-poly <vilib>:"NT Write Value.vi"("Numeric"="T3", "Name"="T3") -> ()  [unwired: 9 in, 1 out]
        n118 = call-poly <vilib>:"NT Write Value.vi"("Numeric"="T4", "Name"="T4") -> ()  [unwired: 9 in, 1 out]
        n119 = call-poly <vilib>:"NT Write Value.vi"("Numeric"="Y1", "Name"="Y1") -> ()  [unwired: 9 in, 1 out]
        n120 = call-poly <vilib>:"NT Write Value.vi"("Numeric"="Y2", "Name"="Y2") -> ()  [unwired: 9 in, 1 out]
      }
    }
  }
  n121 = call "Adjust Dashboard Window.vi"("Sizing Refnums"=w46, "Size Constraints"=w49, "VI"=w57, "WIn Mode"=w32) -> ()  [unwired: 8 in]
  n122 = call "Handle Camera Configuration.vi"("CameraNameRef"=w8, "Camera File Name"="Right", "ClusterRef"=w9) -> ()  [unwired: 9 in]
  n123 = while {
    tunnel: w54 -> [w240]
    tunnel: w33 -> [w238]
    tunnel: [w236] -> _
    tunnel: u32 1000 ("milliseconds to wait") -> [w235]
    tunnel: w24 -> [w229]
    i -> [w236]
    stop <- FALSE stop-if-true
    n124 = local read "Rec Mode"() -> (w231:enum32{"Stop", "Record", "Playback"})
    n125 = Wait on Notification(notifier=w238, timeout in ms (-1)=w235) -> (notification=w237:string, timed out?=w233:bool)  [unwired: 2 in, 2 out]
    n126 = Equal?(x=w231, y=u16 2 ("Rec Mode")) -> (x = y?=w232:bool)
    n127 = Compound Arithmetic op=OR(invert w233, w232) -> (w234:bool)
    n128 = case shown="True" w234 {
      tunnel: w240 -> [_ w243]
      tunnel: w237 -> [_ w242]
      tunnel: w229 -> [_ w241]
      frame False {
      }
      frame True {
        n129 = call <vilib>:"Bind Controls to SmartDashboard.vi"("RPC ref"=w241, "Bound Control Refs"=w243, "Server IP Address"=w242) -> ()  [unwired: 9 in]
      }
    }
  }
  n130 = vi-ref "Playback Controls.vi"() -> (w63:refnum<vi>)
  n131 = property class="VI"() -> ("Panel"=w65:refnum<vi>)  [unwired: 2 in, 2 out]
  n132 = property class="Pnl"(reference=w65) -> ("Panes[]"=w66:refnum<vi>[])  [unwired: 1 in, 2 out]
  n133 = Index Array(array=w66) -> (element=w64:refnum<vi>)  [unwired: 1 in]
  n134 = control-ref of="Test Tree"() -> (w67:refnum<vi>)
  n135 = while {
    tunnel: [w253] -> _
    tunnel: w67 -> [w252]
    tunnel: w63 -> [w251]
    tunnel: w62 -> [w250]
    tunnel: w61 -> [_]
    tunnel: w57 -> [w249]
    tunnel: w24 -> [w248]
    tunnel: w22 -> [w247]
    shift-right: [w246] -> _
    shift-left: _ -> [w245]
    tunnel: w16 -> [w244]
    i -> [w253]
    stop <- FALSE stop-if-true
    n136 = event shown="[0] Timeout" {
      selector: w250 -> [_ _ _ _ _ _ _ _ _ _ _ _ _ _ _ _ _ _ _ _ _]
      dyn-events: [_ _ _ _ _ _ _ _ _ _ _ _ _ _ _ _ w509 _ _ _ _] -> _
      timeout: u32 60 ("milliseconds to wait") -> [_ _ _ _ _ _ _ _ _ _ _ _ _ _ _ _ _ _ _ _ _]
      tunnel: w252 -> [w265 _ _ _ _ _ _ _ _ _ _ _ _ _ _ _ _ _ _ _ _]
      tunnel: "Test Tree" -> [_ _ _ _ _ _ _ _ _ _ _ w476 w484 w486 w490 w498 _ _ _ _ _]
      tunnel: w251 -> [_ _ _ _ _ _ _ _ _ _ _ _ _ _ _ _ w511 _ w529 _ _]
      tunnel: w249 -> [_ _ _ _ _ _ _ _ _ _ _ _ _ _ _ _ w507 _ _ _ _]
      tunnel: w248 -> [_ _ _ _ _ _ _ _ _ _ _ _ _ _ _ _ w503 _ _ _ _]
      tunnel: w247 -> [w260 _ _ _ _ _ w427 _ _ _ _ _ _ _ _ _ _ _ _ _ _]
      tunnel: [w259 w304 w406 w411 w420 w424 w425 w434 w444 w451 w463 w475 w482 w485 w489 w497 w502 w524 w526 w530 w541] -> w246
      tunnel: w245 -> [w259 w304 w406 w411 w420 w424 w425 _ _ w451 w463 w475 w482 w485 w489 w497 w502 w524 w526 w530 w541]
      tunnel: w244 -> [w257 _ _ _ _ _ _ _ _ _ _ _ _ _ _ _ _ _ _ _ _]
      event Timeout {
        n137 = event-data() -> ()  [unwired: 1 in, 1 out]
        n138 = local read "Mode"() -> (w262:T5)
        n139 = case shown="\"Basic\"" "Dashboard Tab" {
          tunnel: w265 -> [_ _ w281 _ _]
          tunnel: "/TestMode/Automatic/" ("Name Pattern") -> [_ _ w280 _ _]
          tunnel: T18 [{"Operation"=enum."Clear", "Color Box"=14013909}, {"Operation"=enum."Clear", "Color Box"=14013909}, {"Operation"=enum."Clear", "Color Box"=14013909}, {"Operation"=enum."Clear", "Color Box"=14013909}, {"Operation"=enum."Update", "Color Box"=14013909}, {"Operation"=enum."Update", "Color Box"=16777215}, {"Operation"=enum."Clear", "Color Box"=14013909}, {"Operation"=enum."Clear", "Color Box"=14013909}, {"Operation"=enum."Clear", "Color Box"=14013909}] -> [_ _ w273 _ w297]
          tunnel: w262 -> [_ _ w272 _ w296]
          tunnel: u32[] [15790320, 15790320, 15790320, 15790320, 16777215, 16777215, 15790320, 15790320, 15790320] -> [_ _ _ _ w302]
          tunnel: w260 -> [_ _ _ _ w290]
          tunnel: w257 -> [_ w267 _ _ _]
          frame "Custom", Default {
          }
          frame "Basic" {
            n140 = call <vilib>:"WPI_DashboardUpdateNames.vi"("Controls on Tab"=w267) -> ()  [unwired: 11 in]
          }
          frame "Test" {
            w279 = -2 ("Active Item:Row Number")
            n141 = Index Array(array=w273, index=w272) -> (element=w274:T21)
            n142 = Unbundle(w274) -> ("Operation"=w275:enum16{"Update", "Clear"}, "Color Box"=w276:u32)
            n143 = call <vilib>:"NT Read String.vi"("Name"="/TestMode/TestName") -> ("String"=w270:string)  [unwired: 9 in, 1 out]
            n144 = call <vilib>:"NT Read and Format Entries as Tree.vi"("Operation"=w275, "Name Pattern"=w280, "Tree Refnum"=w281) -> ()  [unwired: 7 in, 2 out]
            n145 = case shown="\"\"" w270 {
              tunnel: "/TestMode/TestProgress" ("Name") -> [w283 _]
              tunnel: "/TestMode/TestProgressText" ("Name") -> [w282 _]
              frame Default {
                n146 = call <vilib>:"NT Read Number.vi"("Name"=w283) -> ("Numeric"=w284:dbl)  [unwired: 9 in, 1 out]
                n147 = call <vilib>:"NT Read String.vi"("Name"=w282) -> ("String"=w285:string)  [unwired: 9 in, 1 out]
                n148 = Bundle("Numeric"=w284, "String"=w285) -> (→"Progress":cluster{"Numeric":dbl, "String":string})  [unwired: 1 in]
              }
              frame "" {
                n149 = property on="Progress" class="Clust (strict)"("Visible"=FALSE) -> ()  [unwired: 2 in, 2 out]
                n150 = local write "Test Name"(u16 0) -> ()
              }
            }
            n151 = property on="Test Tree" class="Tree (strict)"("Active Item Row Number"=w279, "ActiveColNum"=w279, "CellBG"=w276, "Active Item Row Number"=-1 ("Active Item:Row Number"), "CellBG"=u32 5789784 ("Color Box")) -> ()  [unwired: 2 in, 2 out]
          }
          frame "Variables" {
            n152 = control-ref of="Tree"() -> (w289:refnum<vi>)
            n153 = call <vilib>:"NT Read and Format Entries as Tree.vi"("Tree Refnum"=w289) -> ()  [unwired: 9 in, 2 out]
          }
          frame "Commands" {
            w298 = u32 5789784 ("Color Box")
            w299 = T22 {"Row"=-1, "Column"=-2} ("Active Cell:Active Cell")
            w301 = T22 {"Row"=-2, "Column"=-2} ("Active Cell:Active Cell")
            n154 = Index Array(array=w302, index=w296) -> (element=w300:u32)
            n155 = Index Array(array=w297, index=w296) -> (element=w295:T21)
            n156 = Unbundle(w295) -> ("Operation"=w294:enum16{"Update", "Clear"})  [unwired: 1 out]
            n157 = local read "Command Selection"() -> (w293:i32)
            n158 = property on="Command Selection" class="MCListbox (strict)"("ActiveCell"=w301, "CellBG"=w300, "ActiveCell"=w299, "CellBG"=w298) -> ()  [unwired: 2 in, 2 out]
            n159 = call <vilib>:"WPI_DashboardUpdate RPC Info.vi"("Operation"=w294) -> ("update"=w292:bool, "commands"=w291:string[][])  [unwired: 9 in]
            n160 = property on="Command Selection" class="MCListbox (strict)"("ItemNames"=w291) -> ()  [unwired: 2 in, 2 out]
            n161 = property on="Command Params" class="Tbl (strict)"("Active Cell"=w301, "Cell BG Color"=w300, "Active Cell"=w299, "Cell BG Color"=w298) -> ()  [unwired: 2 in, 2 out]
            n162 = call <vilib>:"WPI_DashboardUpdate Command Params.vi"("Update"=w292, "NewVal"=w293, "Commands"=w291, "Param Tbl"=w290) -> ()  [unwired: 7 in, 1 out]
          }
        }
        n163 = call <vilib>:"Connextion Info.vi"() -> ("Connected"=→"NT Connection":bool)  [unwired: 10 in, 1 out]
      }
      event "Test Tree": Value Change {
        # "Show appropriate\ncontrols"
        n164 = event-data() -> ("CtlRef"=w307:refnum<vi>, "NewVal"=w305:string)  [unwired: 1 in]
        n165 = call <vilib>:"WPI_UtilitiesGetTreeIOName.vi"("NewVal"=w305, "TreeControl in"=w307) -> ("I/O Name"=w308:string)  [unwired: 9 in]
        n166 = case shown="\"Camera\"" w308 {
          selector: w308 -> [_ w315 _ w337 w346 _]
          tunnel: w305 -> [_ _ w334 w336 _ w353]
          tunnel: cluster{string[]}[] [{["640x480", "320x240", "160x120"]}, {["Auto", "Fixed indoor", "Fixed outdoor 1", "Fixed outdoor 2", "Fixed fluorescent 1", "Fixed fluorescent 2", "Hold current"]}, {["Auto", "Flicker-free 50 Hz", "Flicker-free 60 Hz", "Hold current"]}, {["None", "Prioritize frame rate", "Prioritize image quality"]}, {["Monochrome", "Color"]}] -> [_ _ _ _ _ w352]
          frame Default {
            w310 = FALSE ("Visible")
            w309 = FALSE ("Visible")
            n167 = property on="Motor" class="Clust (strict)"("Visible"=w309) -> ()  [unwired: 2 in, 2 out]
            n168 = property on="Test Ring" class="Ring (strict)"("Visible"=w309) -> ()  [unwired: 2 in, 2 out]
            n169 = property on="Rev/Fwd" class="Clust (strict)"("Visible"=w310) -> ()  [unwired: 2 in, 2 out]
            n170 = property on="On/Off" class="Bool (strict)"("Visible"=w310) -> ()  [unwired: 2 in, 2 out]
            n171 = property on="Test Slider" class="Slide (strict)"("Visible"=w310) -> ()  [unwired: 2 in, 2 out]
          }
          frame "Analog Out", "Motor", "PWM" {
            w316 = FALSE ("Visible")
            n172 = case shown="\"Analog Out\"" w315 {
              tunnel: [1.0 ("Value") -1.0 ("Value") 0.0 ("Value")] -> w314
              tunnel: [255.0 ("Value") 1.0 ("Value") 5.0 ("Value")] -> w313
              tunnel: [128.0 ("Value") 0.0 ("Value") 0.0 ("Value")] -> w312
              tunnel: [64.0 ("Value") 0.5 ("Value") 1.0 ("Value")] -> w311
              frame "PWM" {
              }
              frame "Motor", Default {
              }
              frame "Analog Out" {
              }
            }
            n173 = property on="Motor" class="Clust (strict)"("Visible"=TRUE) -> ()  [unwired: 2 in, 2 out]
            n174 = property on="Value" class="Slide (strict)"("Value"=w312, "Scale.Minimum"=w314, "Scale.Maximum"=w313, "Scale.Increment"=w311) -> ()  [unwired: 2 in, 2 out]
            n175 = property on="On/Off" class="Bool (strict)"("Visible"=w316) -> ()  [unwired: 2 in, 2 out]
            n176 = property on="Test Slider" class="Slide (strict)"("Visible"=w316) -> ()  [unwired: 2 in, 2 out]
            n177 = property on="Test Ring" class="Ring (strict)"("Visible"=w316) -> ()  [unwired: 2 in, 2 out]
            n178 = property on="Rev/Fwd" class="Clust (strict)"("Visible"=w316) -> ()  [unwired: 2 in, 2 out]
          }
          frame "Servo" {
            w332 = FALSE ("Visible")
            n179 = call <vilib>:"NT Read Number.vi"("Name"=w334) -> ("Numeric"=w333:dbl)  [unwired: 9 in, 1 out]
            n180 = property on="Test Slider" class="Slide (strict)"("Visible"=TRUE, "Scale.Maximum"=170.0 ("Scale.Range:Maximum")) -> ()  [unwired: 2 in, 2 out]
            n181 = local write "Test Slider"(w333) -> ()
            n182 = property on="Motor" class="Clust (strict)"("Visible"=w332) -> ()  [unwired: 2 in, 2 out]
            n183 = property on="Rev/Fwd" class="Clust (strict)"("Visible"=w332) -> ()  [unwired: 2 in, 2 out]
            n184 = property on="On/Off" class="Bool (strict)"("Visible"=w332) -> ()  [unwired: 2 in, 2 out]
            n185 = property on="Test Ring" class="Ring (strict)"("Visible"=w332) -> ()  [unwired: 2 in, 2 out]
          }
          frame "Relay", "Solenoid" {
            w335 = FALSE ("Visible")
            n186 = property on="Motor" class="Clust (strict)"("Visible"=w335) -> ()  [unwired: 2 in, 2 out]
            n187 = property on="Test Slider" class="Slide (strict)"("Visible"=w335) -> ()  [unwired: 2 in, 2 out]
            n188 = Search and Replace String(input string=w336, search string="/Value  **", replace string="/Direction") -> (result string=w342:string)  [unwired: 5 in, 3 out]
            n189 = property on="Test Ring" class="Ring (strict)"("Visible"=w335) -> ()  [unwired: 2 in, 2 out]
            n190 = call <vilib>:"NT Read String.vi"("Name"=w342) -> ("String"=w340:string)  [unwired: 9 in, 1 out]
            n191 = Equal?(x="Both directions", y=w340) -> (x = y?=w338:bool)
            n192 = Not(x=w338) -> (.not. x?=w339:bool)
            n193 = property on="Rev/Fwd" class="Clust (strict)"("Visible"=w338) -> ()  [unwired: 2 in, 2 out]
            n194 = property on="On/Off" class="Bool (strict)"("Visible"=w339, "Caption.Text"=w337) -> ()  [unwired: 2 in, 2 out]
          }
          frame "Compressor", "Digital Out" {
            w345 = FALSE ("Visible")
            # "Get direction and finish"
            n195 = property on="Motor" class="Clust (strict)"("Visible"=w345) -> ()  [unwired: 2 in, 2 out]
            n196 = property on="Test Slider" class="Slide (strict)"("Visible"=w345) -> ()  [unwired: 2 in, 2 out]
            n197 = property on="Test Ring" class="Ring (strict)"("Visible"=w345) -> ()  [unwired: 2 in, 2 out]
            n198 = property on="On/Off" class="Bool (strict)"("Visible"=TRUE, "Caption.Text"=w346) -> ()  [unwired: 2 in, 2 out]
            n199 = property on="Rev/Fwd" class="Clust (strict)"("Visible"=FALSE) -> ()  [unwired: 2 in, 2 out]
          }
          frame "Camera" {
            n200 = call <vilib>:"Get Last Path Segment.vi"("String in"=w353) -> ("String out"=w354:string)  [unwired: 10 in]
            n201 = property on="On/Off" class="Bool (strict)"("Visible"=FALSE) -> ()  [unwired: 2 in, 2 out]
            n202 = property on="Motor" class="Clust (strict)"("Visible"=FALSE) -> ()  [unwired: 2 in, 2 out]
            n203 = property on="Rev/Fwd" class="Clust (strict)"("Visible"=FALSE) -> ()  [unwired: 2 in, 2 out]
            n204 = case shown="\"White Balance  **\"" w354 {
              tunnel: w353 -> [w360 w369 w378 w387 w396 _ w402]
              tunnel: w352 -> [w358 w366 w375 w384 w393 _ _]
              frame "Size  **" {
                n205 = Index Array(array=w358) -> (element=w357:cluster{string[]})  [unwired: 1 in]
                n206 = call <vilib>:"NT Read String.vi"("Name"=w360) -> ("String"=w359:string)  [unwired: 9 in, 1 out]
                n207 = Unbundle(w357) -> (w355:string[])
                n208 = Match First String(2:w355, 3:w359) -> (0:w356:i32)  [unwired: 1 out]
                n209 = property on="Test Ring" class="Ring (strict)"("Value"=w356, "Strings []"=w355) -> ()  [unwired: 2 in, 2 out]
                n210 = property on="Test Ring" class="Ring (strict)"("Visible"=TRUE) -> ()  [unwired: 2 in, 2 out]
                n211 = property on="Test Slider" class="Slide (strict)"("Visible"=FALSE) -> ()  [unwired: 2 in, 2 out]
              }
              frame "White Balance  **" {
                n212 = Index Array(array=w366, index=1) -> (element=w367:cluster{string[]})
                n213 = call <vilib>:"NT Read String.vi"("Name"=w369) -> ("String"=w368:string)  [unwired: 9 in, 1 out]
                n214 = Unbundle(w367) -> (w364:string[])
                n215 = Match First String(2:w364, 3:w368) -> (0:w363:i32)  [unwired: 1 out]
                n216 = property on="Test Ring" class="Ring (strict)"("Value"=w363, "Strings []"=w364) -> ()  [unwired: 2 in, 2 out]
                n217 = property on="Test Ring" class="Ring (strict)"("Visible"=TRUE) -> ()  [unwired: 2 in, 2 out]
                n218 = property on="Test Slider" class="Slide (strict)"("Visible"=FALSE) -> ()  [unwired: 2 in, 2 out]
              }
              frame "Exposure  **" {
                n219 = Index Array(array=w375, index=2) -> (element=w376:cluster{string[]})
                n220 = call <vilib>:"NT Read String.vi"("Name"=w378) -> ("String"=w377:string)  [unwired: 9 in, 1 out]
                n221 = Unbundle(w376) -> (w372:string[])
                n222 = Match First String(2:w372, 3:w377) -> (0:w373:i32)  [unwired: 1 out]
                n223 = property on="Test Ring" class="Ring (strict)"("Value"=w373, "Strings []"=w372) -> ()  [unwired: 2 in, 2 out]
                n224 = property on="Test Ring" class="Ring (strict)"("Visible"=TRUE) -> ()  [unwired: 2 in, 2 out]
                n225 = property on="Test Slider" class="Slide (strict)"("Visible"=FALSE) -> ()  [unwired: 2 in, 2 out]
              }
              frame "Exposure Priority  **" {
                n226 = Index Array(array=w384, index=3) -> (element=w385:cluster{string[]})
                n227 = call <vilib>:"NT Read String.vi"("Name"=w387) -> ("String"=w386:string)  [unwired: 9 in, 1 out]
                n228 = Unbundle(w385) -> (w381:string[])
                n229 = Match First String(2:w381, 3:w386) -> (0:w382:i32)  [unwired: 1 out]
                n230 = property on="Test Ring" class="Ring (strict)"("Value"=w382, "Strings []"=w381) -> ()  [unwired: 2 in, 2 out]
                n231 = property on="Test Ring" class="Ring (strict)"("Visible"=TRUE) -> ()  [unwired: 2 in, 2 out]
                n232 = property on="Test Slider" class="Slide (strict)"("Visible"=FALSE) -> ()  [unwired: 2 in, 2 out]
              }
              frame "Color Enable  **" {
                n233 = Index Array(array=w393, index=4) -> (element=w394:cluster{string[]})
                n234 = call <vilib>:"NT Read String.vi"("Name"=w396) -> ("String"=w395:string)  [unwired: 9 in, 1 out]
                n235 = Unbundle(w394) -> (w390:string[])
                n236 = Match First String(2:w390, 3:w395) -> (0:w391:i32)  [unwired: 1 out]
                n237 = property on="Test Ring" class="Ring (strict)"("Value"=w391, "Strings []"=w390) -> ()  [unwired: 2 in, 2 out]
                n238 = property on="Test Ring" class="Ring (strict)"("Visible"=TRUE) -> ()  [unwired: 2 in, 2 out]
                n239 = property on="Test Slider" class="Slide (strict)"("Visible"=FALSE) -> ()  [unwired: 2 in, 2 out]
              }
              frame Default {
                n240 = property on="Test Ring" class="Ring (strict)"("Visible"=FALSE) -> ()  [unwired: 2 in, 2 out]
                n241 = property on="Test Slider" class="Slide (strict)"("Visible"=FALSE) -> ()  [unwired: 2 in, 2 out]
              }
              frame "Brightness  **", "Color Level  **", "Compression  **", "FPS  **", "Sharpness  **" {
                n242 = call <vilib>:"NT Read Number.vi"("Name"=w402) -> ("Numeric"=w401:dbl)  [unwired: 9 in, 1 out]
                n243 = local write "Test Slider"(w401) -> ()
                n244 = property on="Test Slider" class="Slide (strict)"("Visible"=TRUE, "Scale.Maximum"=100.0 ("Scale.Range:Maximum")) -> ()  [unwired: 2 in, 2 out]
                n245 = property on="Test Ring" class="Ring (strict)"("Visible"=FALSE) -> ()  [unwired: 2 in, 2 out]
              }
            }
          }
        }
        n246 = property on="Progress" class="Clust (strict)"("Visible"=FALSE) -> ()  [unwired: 2 in, 2 out]
      }
      event "Test Name": Mouse Enter {
        # "Populate the ring with the list of tests"
        n247 = event-data() -> ()  [unwired: 1 in, 1 out]
        n248 = call <vilib>:"NT Read String Array.vi"("Name"="/TestMode/TestList") -> ("String Array"=w410:string[])  [unwired: 9 in, 1 out]
        n249 = Build Array (concatenate)("Select the test to run...", w410) -> (w409:string[])
        n250 = property on="Test Name" class="Ring (strict)"("Strings []"=w409) -> ()  [unwired: 2 in, 2 out]
      }
      event "Test Name": Value Change {
        w412 = FALSE ("Visible")
        # "Tell the robot the test name to run"
        n251 = event-data() -> ("NewVal"=w416:u16)  [unwired: 1 in]
        n252 = property on="Test Name" class="Ring (strict)"() -> ("Strings []"=w417:string[])  [unwired: 2 in, 2 out]
        n253 = local write "Progress"(T6 {"Test Progress"=0, "Test Progress Text"=""} ("Progress")) -> ()
        n254 = Index Array(array=w417, index=w416) -> (element=w415:string)
        n255 = call <vilib>:"NT Write String.vi"("String"=w415, "Name"="/TestMode/TestName") -> ()  [unwired: 9 in, 1 out]
        n256 = property on="Progress" class="Clust (strict)"("Visible"=TRUE) -> ()  [unwired: 2 in, 2 out]
        n257 = property on="Motor" class="Clust (strict)"("Visible"=w412) -> ()  [unwired: 2 in, 2 out]
        n258 = property on="Test Slider" class="Slide (strict)"("Visible"=w412) -> ()  [unwired: 2 in, 2 out]
        n259 = property on="On/Off" class="Bool (strict)"("Visible"=w412) -> ()  [unwired: 2 in, 2 out]
        n260 = property on="Rev/Fwd" class="Clust (strict)"("Visible"=w412) -> ()  [unwired: 2 in, 2 out]
        n261 = property on="Test Ring" class="Ring (strict)"("Visible"=w412) -> ()  [unwired: 2 in, 2 out]
      }
      event "Select Auto": Mouse Enter {
        # "Populate the combo box with the list of autonomous options"
        n262 = event-data() -> ()  [unwired: 1 in, 1 out]
        n263 = call <vilib>:"NT Read String Array.vi"("Name"="Auto List") -> ("String Array"=w419:string[])  [unwired: 9 in, 1 out]
        n264 = property on="Select Auto" class="CmbBox"("Strings[]"=w419) -> ()  [unwired: 2 in, 2 out]
      }
      event "Select Auto": Value Change {
        # "User modified the Auto Selection. Write to NT variable so robot knows."
        n265 = event-data() -> ("NewVal"=w422:string)  [unwired: 1 in]
        n266 = call <vilib>:"NT Write String.vi"("String"=w422, "Name"="Auto Selector") -> ()  [unwired: 9 in, 1 out]
      }
      event "Command Selection": Value Change {
        # "Get the params and show in table"
        n267 = event-data() -> ("NewVal"=w428:i32)  [unwired: 1 in]
        n268 = property on="Command Selection" class="MCListbox (strict)"() -> ("ItemNames"=w426:string[][])  [unwired: 2 in, 2 out]
        n269 = call <vilib>:"WPI_DashboardUpdate Command Params.vi"("NewVal"=w428, "Commands"=w426, "Param Tbl"=w427) -> ()  [unwired: 8 in, 1 out]
      }
      event "Execute Command": Value Change {
        # "Started one, Unique ID holds\nresponse"
        n270 = event-data() -> ()  [unwired: 1 in, 1 out]
        n271 = property on="Command Selection" class="MCListbox (strict)"() -> ("ItemNames"=w439:string[][])  [unwired: 2 in, 2 out]
        n272 = Index Array(array=w439, index (row)="Command Selection", index (col)=0) -> (element=w437:string)
        n273 = call <vilib>:"Invoke Commands.vi"("Command Params"="Command Params", "Function Name"=w437) -> ("Params"=w433:u8, "Started"=w432:bool)  [unwired: 7 in, 1 out]
        n274 = Array Subset(array="Command Params", length (row)=w433) -> (w434:string[][])  [unwired: 3 in]
        n275 = Select(t="Executing" ("Cmd Status"), s=w432, f="" ("Cmd Status")) -> (s? t:f=→"Cmd Status":string)
      }
      event "Command Selection": Double Click {
        n276 = event-data() -> ("Row"=w447:i32)  [unwired: 1 in]
        n277 = property on="Command Selection" class="MCListbox (strict)"() -> ("ItemNames"=w450:string[][])  [unwired: 2 in, 2 out]
        n278 = local read "Command Params"() -> (w446:string[][])
        n279 = Index Array(array=w450, index (row)=w447, index (col)=0) -> (element=w448:string)
        n280 = call <vilib>:"Invoke Commands.vi"("Command Params"=w446, "Function Name"=w448) -> ("Params"=w445:u8, "Started"=w440:bool)  [unwired: 7 in, 1 out]
        n281 = Array Subset(array=w446, length (row)=w445) -> (w444:string[][])  [unwired: 3 in]
        n282 = Select(t="Executing" ("Cmd Status"), s=w440, f="" ("Cmd Status")) -> (s? t:f=w441:string)
        n283 = local write "Cmd Status"(w441) -> ()
      }
      event "CheckList": Double Click {
        # "Shift clears all"
        # "Update symbols on the listbox"
        n284 = event-data() -> ("PlatMods.Shift"=w452:bool, "Row"=w454:i32)  [unwired: 1 in]
        n285 = case shown="True" w452 {
          tunnel: w454 -> [w458 _]
          tunnel: 1 -> [w457 _]
          frame False {
            n286 = property on="CheckList" class="LstBox (strict)"() -> ("Item Symbols"=w456:i32[])  [unwired: 2 in, 2 out]
            n287 = Replace Array Subset(array=w456, new element=w457, index=w458) -> (w455:i32[])
            n288 = property on="CheckList" class="LstBox (strict)"("Item Symbols"=w455) -> ()  [unwired: 2 in, 2 out]
          }
          frame True {
            w459 = 0 ("Top Row")
            n289 = property on="CheckList" class="LstBox (strict)"() -> ("Number of Rows"=w461:u32)  [unwired: 2 in, 2 out]
            n290 = Initialize Array(0, w461) -> (w460:i32[])
            n291 = property on="CheckList" class="LstBox (strict)"("Top Row"=w459, "Value"=w459, "Item Symbols"=w460) -> ()  [unwired: 2 in, 2 out]
          }
        }
      }
      event "CheckList": Key Down {
        # "Update symbols on the listbox\nLeft and right keys check and uncheck"
        n292 = event-data() -> ("VKey"=w465:T19)  [unwired: 1 in]
        n293 = case shown="\"Left\", \"Right\"" w465 {
          selector: w465 -> [w470 _]
          tunnel: eventvkey."Left" ("VKey") -> [w468 _]
          frame "Left", "Right" {
            n294 = Equal?(x=w468, y=w470) -> (x = y?=w469:bool)
            n295 = Select(t=0, s=w469, f=1) -> (s? t:f=w471:i32)
            n296 = property on="CheckList" class="LstBox (strict)"() -> ("Item Symbols"=w474:i32[])  [unwired: 2 in, 2 out]
            n297 = Replace Array Subset(array=w474, new element=w471, index="CheckList") -> (w473:i32[])
            n298 = property on="CheckList" class="LstBox (strict)"("Item Symbols"=w473) -> ()  [unwired: 2 in, 2 out]
          }
          frame Default {
          }
        }
      }
      event "Motor.Enable": Value Change {
        # "When the test mode otor enable helper is set, update that\ntree row item's value"
        n299 = event-data() -> ("NewVal"=w480:bool)  [unwired: 1 in]
        n300 = Unbundle("Motor") -> ("Value"=w479:dbl)  [unwired: 1 out]
        n301 = Select(t=w479, s=w480, f=0.0) -> (s? t:f=w477:dbl)
        n302 = call <vilib>:"NT Write Number.vi"("Numeric"=w477, "Name"=w476) -> ()  [unwired: 9 in, 1 out]
      }
      event "Test Slider": Value Change {
        # "When the test mode slider helper is set, update that\ntree row item's value"
        n303 = event-data() -> ("NewVal"=w483:dbl)  [unwired: 1 in]
        n304 = call <vilib>:"NT Write Number.vi"("Numeric"=w483, "Name"=w484) -> ()  [unwired: 9 in, 1 out]
      }
      event "On/Off": Value Change {
        # "When the test mode on/off helper value is set, update that\ntree row item's value"
        n305 = event-data() -> ("NewVal"=w488:bool)  [unwired: 1 in]
        n306 = Boolean To (0,1)(Boolean=w488) -> (0, 1=w487:i16)
        n307 = call <vilib>:"NT Write Number.vi"("Numeric"=w487, "Name"=w486) -> ()  [unwired: 9 in, 1 out]
      }
      event "Rev/Fwd": Value Change {
        # "When the test mode helper value for relays is set, update that\ntree row item's value"
        n308 = event-data() -> ("NewVal.Forward"=w496:bool, "NewVal.Reverse"=w495:bool)  [unwired: 1 in]
        n309 = Boolean To (0,1)(Boolean=w496) -> (0, 1=w492:i16)
        n310 = Boolean To (0,1)(Boolean=w495) -> (0, 1=w494:i16)
        n311 = Negate(x=w494) -> (-x=w493:i16)
        n312 = Add(x=w492, y=w493) -> (x+y=w491:i16)
        n313 = call <vilib>:"NT Write Number.vi"("Numeric"=w491, "Name"=w490) -> ()  [unwired: 9 in, 1 out]
      }
      event "Test Ring": Value Change {
        # "When a test mode helper value is selected from the ring,\nset the tree item's variable to the string value"
        n314 = event-data() -> ("NewVal"=w500:u16)  [unwired: 1 in]
        n315 = property on="Test Ring" class="Ring (strict)"() -> ("Strings []"=w501:string[])  [unwired: 2 in, 2 out]
        n316 = Index Array(array=w501, index=w500) -> (element=w499:string)
        n317 = call <vilib>:"NT Write String.vi"("String"=w499, "Name"=w498) -> ()  [unwired: 9 in, 1 out]
      }
      event "Rec Mode": Value Change {
        # "Update globals for recording mode and path to read log from.\nClear when logging and let NetworkTables set path for vision to\nuse."
        n318 = event-data() -> ("NewVal"=w512:enum32{"Stop", "Record", "Playback"})  [unwired: 1 in]
        n319 = global write "WPI_DashboardLogging Global.vi" "Logging Filename"(path "") -> ()
        n320 = global write "WPI_DashboardLogging Global.vi" "Recording"(w512) -> ()
        n321 = case shown="\"Playback\"" w512 {
          tunnel: w511 -> [_ w514 w523]
          tunnel: [_ _ w522] -> w509
          tunnel: [_ _ w521] -> _
          tunnel: w507 -> [_ _ w519]
          tunnel: cluster{i32, i32} {-250, 170} -> [_ _ w518]
          tunnel: [_ _ T20 {"Image Size"=TRUE, "Image Type"=TRUE, "Pixel Value"=TRUE, "ROI Information"=TRUE, "Zoom Factor"=FALSE} ("Image Information Shown:All Elements")] -> w505
          tunnel: [_ _ TRUE ("Zoom Factor")] -> w504
          tunnel: w503 -> [_ _ w515]
          frame Default {
          }
          frame "Stop", "Record" {
            # "Place Window too"
            n322 = invoke class="VI" method="FP.Close"(reference=w514) -> (reference out=w513:refnum<vi>)  [unwired: 2 in, 2 out]
            n323 = invoke class="VI" method="Abort VI"(reference=w513) -> ()  [unwired: 2 in, 3 out]
          }
          frame "Playback" {
            n324 = call "Open Playback Panel.vi"("Offset"=w518, "DB VI Ref"=w519, "Playback in"=w523) -> ("Playback out"=w520:refnum<vi>)  [unwired: 8 in]
            n325 = register-events(w520, w515) -> (reference out=w522:refnum<event-registration>, error out=w521:errorcluster)  [unwired: 2 in]
          }
        }
        n326 = property on="Camera Image" class="ImageControl"("Image Information Shown"=w505, "Image Information Visible"=w504) -> ()  [unwired: 2 in, 2 out]
        n327 = call <vilib>:"WPI_DashboardNT Log FieldName Cache.vi"("Operation"=enum16{"Lookup/Add", "Index", "Clear"}."Clear") -> ()  [unwired: 8 in, 3 out]
      }
      event Panel Close {
        w525 = enum32{"Stop", "Record", "Playback"}."Stop" ("Rec Mode")
        # "Playback window has been closed, abort"
        n328 = event-data() -> ()  [unwired: 1 in, 4 out]
        n329 = local write "Rec Mode"(w525) -> ()
        n330 = global write "WPI_DashboardLogging Global.vi" "Recording"(w525) -> ()
      }
      event Panel Close {
        # "Abort playback window and ourself"
        n331 = event-data() -> ()  [unwired: 1 in, 4 out]
        n332 = invoke class="VI" method="FP.Close"(reference=w529) -> (reference out=w528:refnum<vi>)  [unwired: 2 in, 2 out]
        n333 = invoke class="VI" method="Abort VI"(reference=w528) -> (error out=w527:errorcluster)  [unwired: 2 in, 2 out]
        n334 = invoke class="VI" method="Abort VI"(error in=w527) -> ()  [unwired: 2 in, 3 out]
      }
      event User Event {
        n335 = event-data() -> ("IDs"=w536:cluster{"RPC field ID":u16, "Unique ID":u16}, "String"=w535:string)  [unwired: 1 in]
        n336 = Bundle("IDs"=w536, "String"=w535) -> (w534:T8)  [unwired: 1 in]
        n337 = call <vilib>:"Retrieve RPC Response.vi"("RPC Response"=w534) -> ("Output"=w532:string[][])  [unwired: 10 in]
        n338 = Build Array (concatenate)(w530, w532) -> (w531:string[][])
        n339 = local write "Command Params"(w531) -> ()
        n340 = local write "Cmd Status"("" ("Cmd Status")) -> ()
      }
      event "Tree": Double Click {
        n341 = event-data() -> ("PlatMods"=w540:T23, "Tag"=w539:string)  [unwired: 1 in]
        n342 = Unbundle(w540) -> ("Shift"=w538:bool)  [unwired: 4 out]
        n343 = Not(x=w538) -> (.not. x?=w537:bool)
        n344 = call <vilib>:"NT Update Persistence.vi"("Persistence"=w537, "Name"=w539) -> ()  [unwired: 9 in, 1 out]
      }
    }
  }
  n345 = while {
    tunnel: w64 -> [w543]
    i -> [w546]
    stop <- FALSE stop-if-true
    n346 = Wait (ms)(milliseconds to wait=u32 100) -> ()  [unwired: 1 out]
    n347 = case shown="\"Playback\"" "Rec Mode" {
      tunnel: w546 -> [_ _ w561]
      tunnel: [u32 2829099 ("Base Color") u32 11141120 ("Target Color") w550] -> w542
      frame "Stop", Default {
        # "Reset the color, extra updates don't cost much"
      }
      frame "Record" {
      }
      frame "Playback" {
        # "Playback"
        n348 = Quotient & Remainder(x=w561, y=u32 50 ("milliseconds to wait")) -> (x-y*floor(x/y)=w557:u32)  [unwired: 1 out]
        n349 = Divide(x=w557, y=u32 50 ("milliseconds to wait")) -> (x/y=w554:dbl)
        n350 = Multiply(x=6.283185307179586, y=w554) -> (x*y=w559:dbl)
        n351 = Sine(x=w559) -> (sin(x)=w558:dbl)
        n352 = Absolute Value(x=w558) -> (abs(x)=w551:dbl)
        n353 = call "Interpolate RGB Color.vi"("Proportion"=w551, "Target Color"=u32 30976, "Base Color"=u32 2829099) -> ("Result Color"=w550:u32)  [unwired: 8 in]
      }
    }
    n354 = property class="Pane"(reference=w543, "PaneColor"=w542) -> ()  [unwired: 1 in, 2 out]
  }
  n355 = local write "Dashboard Tab"(T3."Drive" ("Dashboard Tab")) -> ()
  n356 = property on="On/Off" class="Bool (strict)"("Visible"=w34) -> ()  [unwired: 2 in, 2 out]
  n357 = property on="Motor" class="Clust (strict)"("Visible"=w34) -> ()  [unwired: 2 in, 2 out]
  n358 = property on="Progress" class="Clust (strict)"("Visible"=w34) -> ()  [unwired: 2 in, 2 out]
  n359 = property on="Test Ring" class="Ring (strict)"("Visible"=w34) -> ()  [unwired: 2 in, 2 out]
  n360 = property on="Rev/Fwd" class="Clust (strict)"("Visible"=w34) -> ()  [unwired: 2 in, 2 out]
  n361 = local write "Command Selection"(u16 0 ("milliseconds to wait")) -> ()
  n362 = while {
    tunnel: u16 1741 ("timeout ms (25000)") -> [w563]
    stop <- FALSE stop-if-true
    n363 = TCP Create Listener(10:w563) -> (0:w562:errorcluster, 3:w564:refnum<k5>)  [unwired: 4 in, 1 out]
    n364 = case shown="No Error" w562 {
      selector: w562 -> [w566 _]
      tunnel: w564 -> [w567 _]
      frame No Error {
        n365 = while {
          tunnel: w567 -> [w570]
          tunnel: w566 -> [w569]
          stop <- FALSE stop-if-true
          n366 = TCP Wait On Listener(8:w569, 11:w570) -> (0:w571:errorcluster, 4:w572:refnum<k5>)  [unwired: 2 in, 3 out]
          n367 = local write "TCP"(w572) -> ()
          n368 = case shown="No Error" w571 {
            frame No Error {
            }
            frame Error {
              n369 = Wait (ms)(milliseconds to wait=u32 1000) -> ()  [unwired: 1 out]
            }
          }
        }
      }
      frame Error {
        n370 = Wait (ms)(milliseconds to wait=u32 1000) -> ()  [unwired: 1 out]
      }
    }
  }
  n371 = local write "Command Params"(string[][] [] ("Command Params")) -> ()
  n372 = global write "WPI_DashboardLogging Global.vi" "Recording"(w58) -> ()
  n373 = local write "Rec Mode"(w58) -> ()
  n374 = call <vilib>:"NT Write String.vi"("String"="Select Auto", "Name"="Auto Selector") -> ()  [unwired: 9 in, 1 out]
